vi "Events_DELTA.vi"(8 "hearbeat":bool, 10 "time":u32, 11 "responsein":string) -> (3 "responseout":string)   [LabVIEW 2015]
doc: "Definition of all events sent by the SSE server to the clients"
panel:
  # "Events"
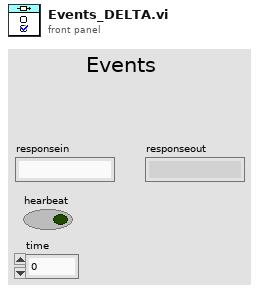
[diagram p1: front panel]
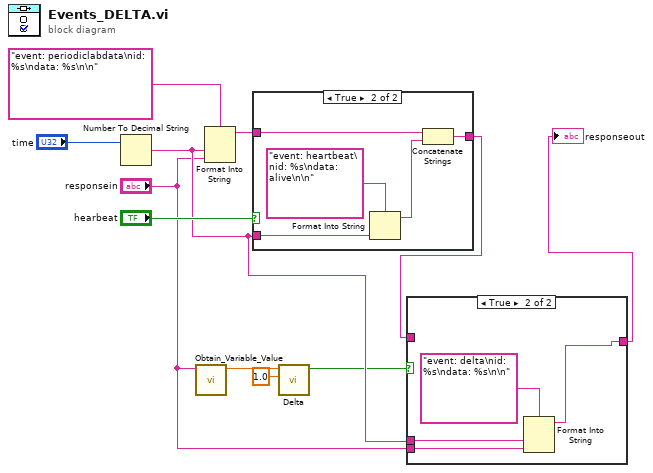
[diagram p0: block diagram]
diagram:
  n1 = Number To Decimal String(number="time") -> (decimal integer string=w4:string)  [unwired: 1 in]
  n2 = call "Obtain_Variable_Value.vi"("JSON result"="responsein") -> ("currentValue"=w7:dbl)  [unwired: 9 in]
  n3 = Format Into String(format string="event: periodiclabdata\nid: %s\ndata: %s\n\n", w4, "responsein") -> (resulting string=w10:string)  [unwired: 2 in, 1 out]
  n4 = case shown="True" "hearbeat" {
    tunnel: [w12 w17] -> w5
    tunnel: w10 -> [w12 w16]
    tunnel: w4 -> [_ w13]
    frame False {
    }
    frame True {
      n5 = Format Into String(format string="event: heartbeat\nid: %s\ndata: alive\n\n", w13) -> (resulting string=w14:string)  [unwired: 2 in, 1 out]
      n6 = Concatenate Strings(w16, w14) -> (w17:string)
    }
  }
  n7 = call "Delta.vi"("currentValue"=w7, "delta"=1.0) -> ("triggerEvent"=w1:bool)  [unwired: 8 in]
  n8 = case shown="True" w1 {
    tunnel: [w18 w19] -> w3
    tunnel: w5 -> [w18 _]
    tunnel: w4 -> [_ w21]
    tunnel: "responsein" -> [_ w20]
    frame False {
    }
    frame True {
      n9 = Format Into String(format string="event: delta\nid: %s\ndata: %s\n\n", w21, w20) -> (resulting string=w19:string)  [unwired: 2 in, 1 out]
    }
  }
  "responseout" <- w3
